vi "Intake_Globals.vi"() -> ()   [LabVIEW 2019]
uses:
  Subsystems/Intake/Intake_Cluster.ctl
panel:
  in  "Intake_Left":string="Intake_Left"
  in  "Intake_Right":string="Intake_Right"
  in  "Intake_Execute_Notifier":refnum<notifier>
  in  "Intake_Set_Notifier":refnum<notifier>
  in  "Intake_Execute_Ref":string="Intake_Execute_Ref"
  in  "Intake_Set_Ref":string="Intake_Set_Ref"
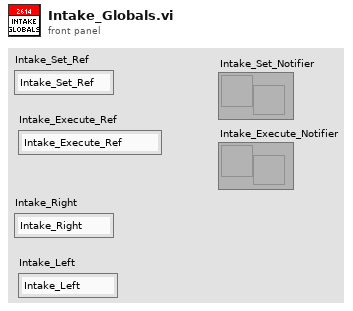
[diagram p1: front panel]
diagram:
